vi "Drive Core.vi"() -> ()   [LabVIEW 2014]
uses:
  <vilib>/Rock Robotics/WPI/DriverStation/WPI_DriverStationRobotMode2.ctl
  Begin/Global Variables.vi
  Begin/Global Constants.vi
  Begin/Global RefNums.vi
panel:
  in  "Reset Encoders":bool
  out "Counts FR":i32
  out "Counts FL":i32
  out "Counts BR":i32
  out "Counts BL":i32
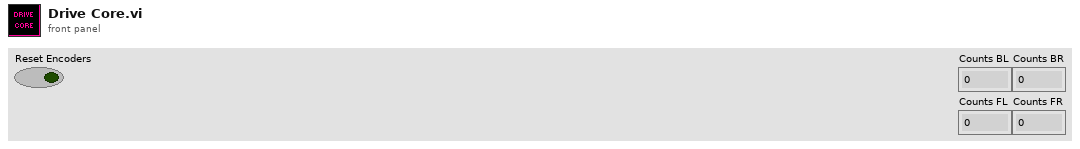
[diagram p1: front panel]
types:
  T1 = typedef "WPI_DriverStationRobotMode2.ctl" = enum16{"Autonomous Disabled", "Autonomous Enabled", "Teleop Disabled", "Teleop Enabled", "Disconnected", "Finish", "Test Disabled", "Test Enabled", "Emergency Stopped"}
  T2 = cluster{"Header P":dbl, "Header I":dbl, "Header D":dbl}
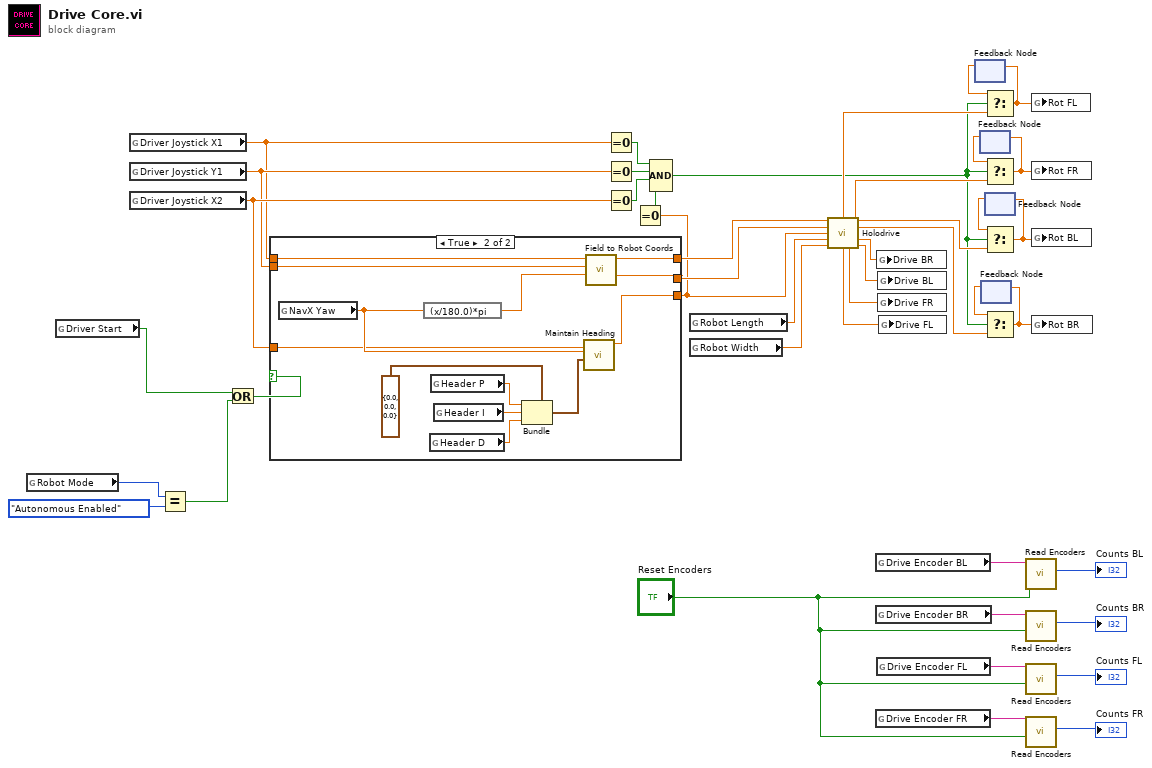
[diagram p0: block diagram]
diagram:
  n1 = global read "Global Variables.vi" "Robot Mode"() -> (w40:T1)
  n2 = global read "Global Variables.vi" "Driver Start"() -> (w12:bool)
  n3 = global read "Global Variables.vi" "Driver Joystick X1"() -> (w36:dbl)
  n4 = global read "Global Variables.vi" "Driver Joystick Y1"() -> (w37:dbl)
  n5 = global read "Global Variables.vi" "Driver Joystick X2"() -> (w41:dbl)
  n6 = Equal?(x=w40, y=WPI_DriverStationRobotMode2."Autonomous Enabled") -> (x = y?=w14:bool)
  n7 = Or(x=w12, y=w14) -> (x .or. y?=w13:bool)
  n8 = case shown="True" w13 {
    tunnel: w36 -> [w46 w59]
    tunnel: w37 -> [w45 w58]
    tunnel: [w46 w57] -> w38
    tunnel: [w45 w56] -> w39
    tunnel: w41 -> [w44 w47]
    tunnel: [w44 w55] -> w10
    frame False {
    }
    frame True {
      n9 = global read "Global Variables.vi" "NavX Yaw"() -> (w49:dbl)
      n10 = expression code="(x/180.0)*pi" ("degrees to radians")(w49) -> (w54:dbl)
      n11 = global read "Global Constants.vi" "Header D"() -> (w51:dbl)
      n12 = global read "Global Constants.vi" "Header P"() -> (w53:dbl)
      n13 = global read "Global Constants.vi" "Header I"() -> (w52:dbl)
      n14 = Bundle(cluster=T2 {"Header P"=0.0, "Header I"=0.0, "Header D"=0.0}, "Header P"=w53, "Header I"=w52, "Header D"=w51) -> (w48:T2)
      n15 = call "Maintain Heading.vi"("PID gains"=w48, "NavX Yaw"=w49, "Raw Driver Joystick X2"=w47) -> ("Driver Joystick X2"=w55:dbl)  [unwired: 8 in]
      n16 = call "Field to Robot Coords.vi"("gyro"=w54, "Joystick y"=w58, "Joystick x"=w59) -> ("robot y"=w56:dbl, "robot x"=w57:dbl)  [unwired: 7 in]
    }
  }
  n17 = Equal To 0?(x=w36) -> (x = 0?=w19:bool)
  n18 = Equal To 0?(x=w37) -> (x = 0?=w20:bool)
  n19 = Equal To 0?(x=w41) -> (x = 0?=w21:bool)
  n20 = Equal To 0?(x=w10) -> (x = 0?=w11:bool)
  n21 = Compound Arithmetic op=AND(w19, w20, w21, w11) -> (w22:bool)
  n22 = global read "Global Constants.vi" "Robot Length"() -> (w42:dbl)
  n23 = global read "Global Constants.vi" "Robot Width"() -> (w43:dbl)
  n24 = call "Holodrive.vi"("Translation X"=w38, "Translation Y"=w39, "Angular"=w10, "Robot Length"=w42, "Robot Width"=w43) -> ("FL Rot"=w28:dbl, "FR Rot"=w25:dbl, "BL Rot"=w26:dbl, "BR Rot"=w27:dbl, "BR Drive"=w18:dbl, "FL Drive"=w15:dbl, "FR Drive"=w16:dbl, "BL Drive"=w17:dbl)  [unwired: 3 in]
  n25 = global read "Global RefNums.vi" "Drive Encoder BL"() -> (w9:string)
  n26 = global read "Global RefNums.vi" "Drive Encoder BR"() -> (w8:string)
  n27 = global read "Global RefNums.vi" "Drive Encoder FR"() -> (w6:string)
  n28 = global write "Global Variables.vi" "Drive BR"(w18) -> ()
  n29 = global read "Global RefNums.vi" "Drive Encoder FL"() -> (w7:string)
  n30 = global write "Global Variables.vi" "Drive BL"(w17) -> ()
  n31 = global write "Global Variables.vi" "Drive FR"(w16) -> ()
  n32 = global write "Global Variables.vi" "Drive FL"(w15) -> ()
  n33 = feedback #1() -> (w30:dbl)  [unwired: 1 in]
  n34 = feedback #2() -> (w24:dbl)  [unwired: 1 in]
  n35 = feedback #3() -> (w34:dbl)  [unwired: 1 in]
  n36 = Select(t=w30, s=w22, f=w28) -> (s? t:f=w29:dbl)
  n37 = feedback-in #1(w29) -> ()
  n38 = Select(t=w24, s=w22, f=w25) -> (s? t:f=w23:dbl)
  n39 = feedback-in #2(w23) -> ()
  n40 = feedback #4() -> (w32:dbl)  [unwired: 1 in]
  n41 = Select(t=w32, s=w22, f=w26) -> (s? t:f=w31:dbl)
  n42 = feedback-in #4(w31) -> ()
  n43 = Select(t=w34, s=w22, f=w27) -> (s? t:f=w33:dbl)
  n44 = feedback-in #3(w33) -> ()
  n45 = call "Read Encoders.vi"("Reset Encoders"="Reset Encoders", "Encoder"=w9) -> ("Counts"=→"Counts BL":i32)  [unwired: 9 in]
  n46 = call "Read Encoders.vi"("Reset Encoders"="Reset Encoders", "Encoder"=w8) -> ("Counts"=→"Counts BR":i32)  [unwired: 9 in]
  n47 = call "Read Encoders.vi"("Reset Encoders"="Reset Encoders", "Encoder"=w7) -> ("Counts"=→"Counts FL":i32)  [unwired: 9 in]
  n48 = call "Read Encoders.vi"("Reset Encoders"="Reset Encoders", "Encoder"=w6) -> ("Counts"=→"Counts FR":i32)  [unwired: 9 in]
  n49 = global write "Global Variables.vi" "Rot FL"(w29) -> ()
  n50 = global write "Global Variables.vi" "Rot FR"(w23) -> ()
  n51 = global write "Global Variables.vi" "Rot BL"(w31) -> ()
  n52 = global write "Global Variables.vi" "Rot BR"(w33) -> ()
